vi "rpc_tsmaster_create_client.vi"(8 "error in (no error)":errorcluster caption="Incorrect input (no errors)", 10 "AppName":string="LABFD", 11 "Path input":path) -> (0 "error output":errorcluster, 1 "AHandle":i32, 2 "return":i32, 3 "Path output":path)   [LabVIEW 2014]
doc: "Function introduction: Create a TSMaster Rpc client\nAfter calling the location to initialize the tsmaster lib library\nInput parameter ATSMasterAppName: TSMaster server-side application name;\nAHHandle: TSMaster Rpc Client Handle\nReturn value==0: Function execution successful\nOther values: Function execution failed"
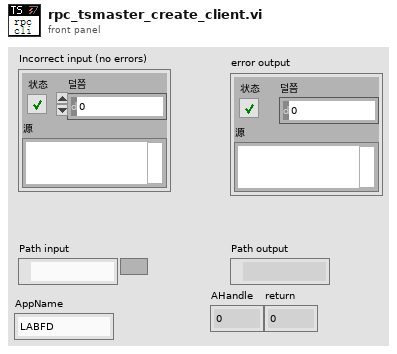
[diagram p1: front panel]
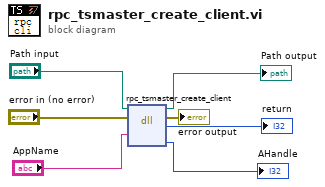
[diagram p0: block diagram]
diagram:
  n1 = dll-call lib="D:/Program Files (x86)/TOSUN/TSMaster/bin/TSMaster.dll" fn="rpc_tsmaster_create_client"(path in="Path input", error in="error in (no error)", "ATSMasterAppName"="AppName") -> (path out=→"Path output":path, error out=→"error output":errorcluster, "return"=→"return":i32, "AHandle"=→"AHandle":i32)  [unwired: 3 in]
